vi "Micron Optics sm130 Streaming Peak Wavelength.vi"() -> ()   [LabVIEW 2015]
doc: "Puts the instrument into streaming mode and graphs the peak wavelengths from the device against time."
uses:
  Micron Optics sm130.lvlib
panel:
  in  "Stop":bool
  in  "CH4 Sensor Number (1)":i32=1
  in  "CH3 Sensor Number (1)":i32=1
  in  "CH2 Sensor Number (1)":i32=1
  in  "CH1 Sensor Number (1)":i32=1
  out "Channel 4":dbl(graph)
  out "Channel 3":dbl(graph)
  out "Channel 2":dbl(graph)
  out "Channel 1":dbl(graph)
  in  "Sample Rate (1000 Hz)":i32=1000
  in  "VISA resource name":refnum<visa-resource-name>
  # "(c) 2012 National Instruments.  ALL RIGHTS RESERVED."
  # "Sensor Number"
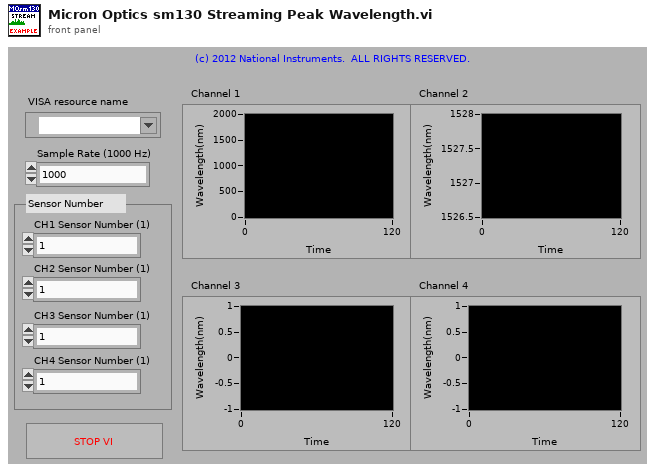
[diagram p1: front panel]
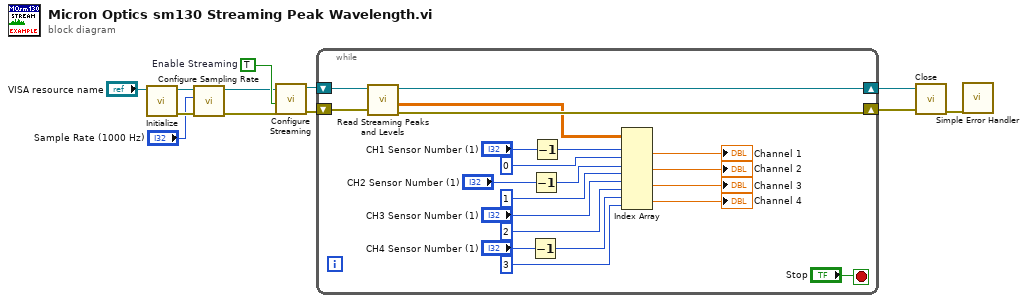
[diagram p0: block diagram]
diagram:
  w9 = TRUE  # Enable Streaming
  n1 = call "Initialize.vi"("VISA resource name"="VISA resource name") -> ("error out"=w5:errorcluster, "VISA resource name out"=w6:refnum<visa-resource-name>)  [unwired: 9 in]
  n2 = call "Configure Sampling Rate.vi"("error in (no error)"=w5, "Sample Rate (1000 Hz)"="Sample Rate (1000 Hz)", "VISA resource name"=w6) -> ("error out"=w4:errorcluster, "VISA resource name out"=w3:refnum<visa-resource-name>)  [unwired: 7 in]
  n3 = call "Configure Streaming.vi"("error in (no error)"=w4, "Enable Streaming (Enable)"=w9, "VISA resource name"=w3) -> ("error out"=w7:errorcluster, "VISA resource name out"=w8:refnum<visa-resource-name>)  [unwired: 7 in]
  n4 = while {
    shift-right: [w15] -> w11
    shift-left: w7 -> [w16]
    shift-right: [w18] -> w12
    shift-left: w8 -> [w17]
    stop <- "Stop" stop-if-true
    n5 = call "Read Streaming Peaks and Levels.vi"("error in (no error)"=w16, "VISA resource name"=w17) -> ("error out"=w15:errorcluster, "Peak Wavelengths (nm)"=w14:dbl[][], "VISA resource name out"=w18:refnum<visa-resource-name>)  [unwired: 5 in, 2 out]
    n6 = Decrement(x="CH4 Sensor Number (1)") -> (x-1=w28:i32)
    n7 = Decrement(x="CH2 Sensor Number (1)") -> (x-1=w26:i32)
    n8 = Decrement(x="CH1 Sensor Number (1)") -> (x-1=w25:i32)
    n9 = Index Array(array=w14, index (row) #1=w25, index (col) #1=0 ("disabled index (col)"), index (row) #2=w26, index (col) #2=1 ("index (col)"), index (row) #3="CH3 Sensor Number (1)", index (col) #3=2 ("index (col)"), index (row) #4=w28, index (col) #4=3 ("index (col)")) -> (element #1=→"Channel 1":dbl, element #2=→"Channel 2":dbl, element #3=→"Channel 3":dbl, element #4=→"Channel 4":dbl)
  }
  n10 = call "Close.vi"("error in (no error)"=w11, "VISA resource name"=w12) -> ("error out"=w1:errorcluster)  [unwired: 9 in]
  n11 = call <vilib>:"Simple Error Handler.vi"("error in (no error)"=w1) -> ()  [unwired: 4 in, 5 out]
